vi "VisaBasicForS2Tool.vi"(1 "VISA resource name":refnum<visa-resource-name>, 2 "Cmd":string, 3 "TimeOut":bool=TRUE, 4 "Time(0.1)":u32=10, 5 "error in (no error)":errorcluster, 8 "VisaAction":enum16{"Open", "Send", "Recieve", "Close"}(ring)) -> (16 "read string":string, 19 "error out":errorcluster)   [LabVIEW 2019]
uses:
  <vilib>/Instr/_visa.llb/VISA Configure Serial Port (Instr).vi
  LLB/Commonly VI.lvlib
panel:
  out "Numeric":i32
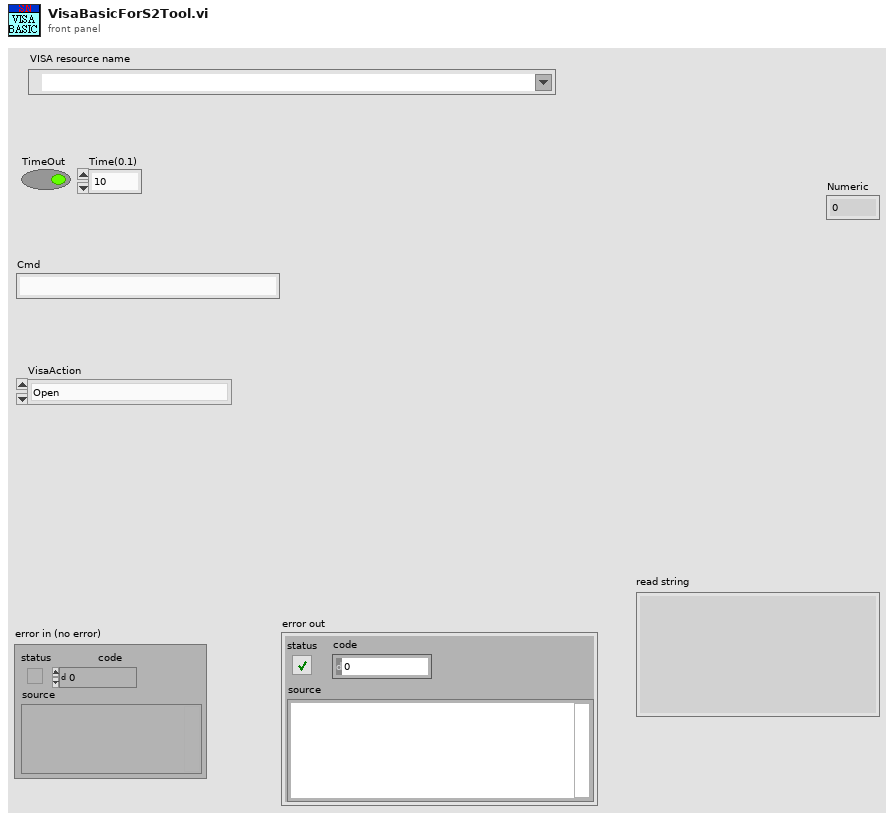
[diagram p1: front panel]
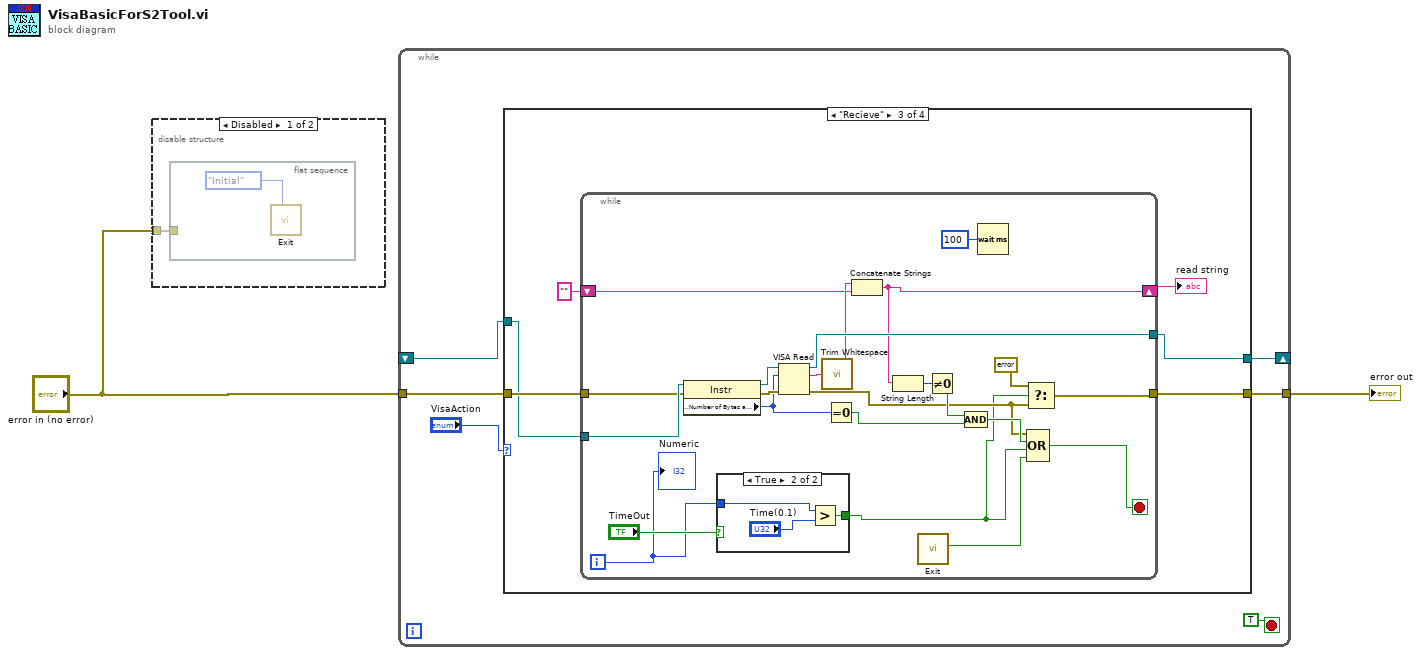
[diagram p0: block diagram]
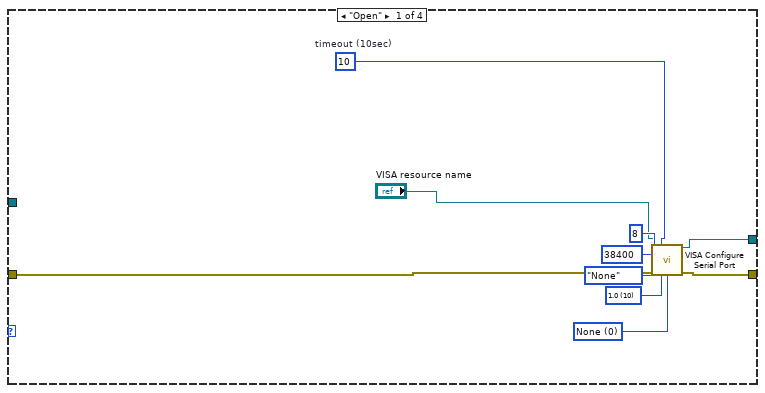
[diagram p3: hidden frame]
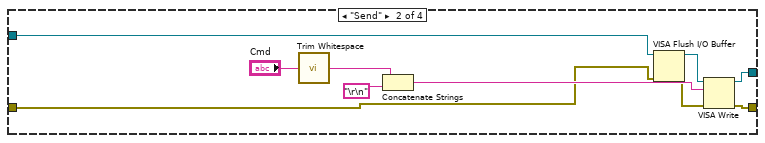
[diagram p4: hidden frame]
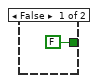
[diagram p5: hidden frame]
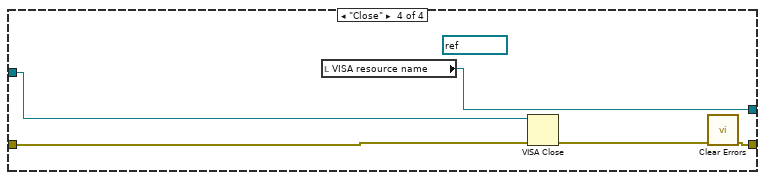
[diagram p6: hidden frame]
diagram:
  n1 = disable-structure shown="Disabled" {
    disable-tunnel: "error in (no error)" -> [w3 _]
    frame Disabled {
      n2 = flat-sequence {
        tunnel: w3 -> [_]
        frame #0 {
          n3 = call "Exit.vi"("Enum"=enum16{"Initial", "Read", "Write"}."Initial") -> ()  [unwired: 10 in, 1 out]
        }
      }
    }
    frame Enabled {
    }
  }
  n4 = while {
    tunnel: "error in (no error)" -> [w8]
    tunnel: [w9] -> w1
    shift-right: [w6] -> _
    shift-left: _ -> [w5]
    stop <- TRUE stop-if-true
    n5 = case shown="\"Recieve\"" "VisaAction" {
      tunnel: [w20 w30 w35 w65] -> w9
      tunnel: w8 -> [w19 w21 w36 w67]
      tunnel: w5 -> [_ w22 w32 w66]
      tunnel: [w12 w25 w31 w64] -> w6
      frame "Open" {
        w14 = u16 0 items=["None", "XON/XOFF", "RTS/CTS", "XON/XOFF & RTS/CTS", "DTR/DSR", "XON/XOFF & DTR/DSR"] ("flow control (0:none)")
        w15 = u16 10 items=["1.0"=10, "1.5"=15, "2.0"=20] ("stop bits (10: 1 bit)")
        w18 = u32 10  # timeout (10sec)
        n6 = call-poly "VISA Configure Serial Port"("VISA resource name"="VISA resource name", "timeout (10sec)"=w18, "baud rate (9600)"=u32 38400, "data bits (8)"=u16 8, "parity (0:none)"=enum16{"None", "Odd", "Even", "Mark", "Space"}."None", "error in (no error)"=w19, "stop bits (10: 1 bit)"=w15, "flow control (0:none)"=w14) -> ("VISA resource name out"=w12:refnum<visa-resource-name>, "error out"=w20:errorcluster)  [unwired: 1 in, 5 out]
      }
      frame "Send" {
        n7 = call <vilib>:"Trim Whitespace.vi"("string"="Cmd") -> ("trimmed string"=w26:string)  [unwired: 1 in]
        n8 = Concatenate Strings(w26, "\r\n") -> (w27:string)
        n9 = VISA Flush I/O Buffer(VISA resource name=w22, error in (no error)=w21) -> (VISA resource name out=w23:refnum<visa-resource-name>, error out=w24:errorcluster)  [unwired: 1 in]
        n10 = VISA Write(VISA resource name=w23, write buffer=w27, error in (no error)=w24) -> (VISA resource name out=w25:refnum<visa-resource-name>, error out=w30:errorcluster)  [unwired: 1 out]
      }
      frame "Recieve" {
        n11 = while {
          tunnel: w32 -> [w57]
          tunnel: w36 -> [w56]
          tunnel: [w55] -> w31
          tunnel: [w50] -> w35
          shift-right: [w47] -> w34
          shift-left: "" ("trimmed string") -> [w53]
          i -> [w38]
          stop <- w51 stop-if-true
          n12 = property class="Instr"(reference=w57, error in=w56) -> (reference out=w58:refnum<visa-resource-name>, error out=w59:errorcluster, "Serial Settings:Number of Bytes at Serial Port"=w39:u32)
          n13 = case shown="True" "TimeOut" {
            tunnel: w38 -> [_ w63]
            tunnel: [FALSE w61] -> w37
            frame False {
            }
            frame True {
              n14 = Greater?(x=w63, y="Time(0.1)") -> (0:w61:bool)
            }
          }
          n15 = VISA Read(VISA resource name=w58, byte count=w39, error in (no error)=w59) -> (VISA resource name out=w55:refnum<visa-resource-name>, read buffer=w41:string, error out=w43:errorcluster)  [unwired: 1 out]
          n16 = call <vilib>:"Trim Whitespace.vi"("string"=w41) -> ("trimmed string"=w54:string)  [unwired: 1 in]
          n17 = Equal To 0?(x=w39) -> (x = 0?=w48:bool)
          n18 = Concatenate Strings(w53, w54) -> (w47:string)
          n19 = String Length(string=w47) -> (length=w46:i32)
          n20 = call "Exit.vi"() -> ("ExitOut"=w42:bool)  [unwired: 11 in]
          n21 = Not Equal To 0?(x=w46) -> (x != 0?=w45:bool)
          n22 = Compound Arithmetic op=AND(w45, w48) -> (w44:bool)
          n23 = Wait (ms)(milliseconds to wait=u32 100) -> ()  [unwired: 1 out]
          n24 = Select(t=errorcluster {"status"=TRUE, "code"=11312, "source"=""}, s=w37, f=w43) -> (s? t:f=w50:errorcluster)
          n25 = Compound Arithmetic op=OR(w43, w44, w37, w42) -> (w51:bool)
          "Numeric" <- w38
        }
        "read string" <- w34
      }
      frame "Close" {
        (unwired) refnum<visa-resource-name> "COM3" ("VISA resource name out")
        n26 = local read "VISA resource name"() -> (w64:refnum<visa-resource-name>)
        n27 = VISA Close(VISA resource name=w66, error in (no error)=w67) -> (error out=w68:errorcluster)
        n28 = call <vilib>:"Clear Errors.vi"("error in (no error)"=w68) -> ("error out"=w65:errorcluster)  [unwired: 5 in, 1 out]
      }
    }
  }
  "error out" <- w1
